vi "Is Nominal State.vi"(11 "Base jettl in":refnum<class "Base jettl.lvclass">) -> (2 "Is Nominal State?":bool)   [LabVIEW 2021, in "jettl.lvlib" / "Base jettl.lvclass"]
uses:
  Base jettl.lvclass
  State.ctl
  Base jettl.lvclass/Base jettl.ctl
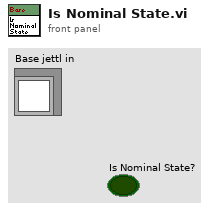
[diagram p1: front panel]
types:
  T1 = typedef "jettl.lvlib/Base jettl.lvclass/State.ctl" = enum16{"Nominal", "Teardown", "Error"}
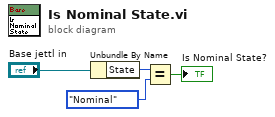
[diagram p0: block diagram]
diagram:
  n1 = Unbundle By Name("Base jettl in") -> ("State"=w2:T1)
  n2 = Equal?(x=w2, y=State."Nominal") -> (x = y?=→"Is Nominal State?":bool)
